vi "采配水仪器参数改变发送 (子VI).vi"(8 "错误输入":errorcluster caption="错误输出") -> (0 "错误输出":errorcluster)   [LabVIEW 2016, in "数据传输系统-03.lvlib"]
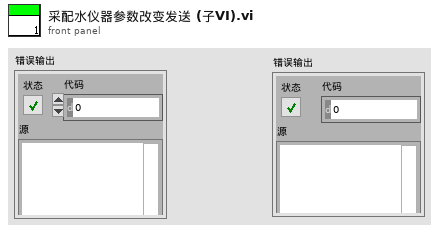
[diagram p1: front panel]
types:
  T1 = cluster{"CODMn关键参数":bool, "氨氮关键参数":bool, "总磷关键参数":bool, "总氮关键参数":bool, "CODCr关键参数":bool, "采配水关键参数":bool}
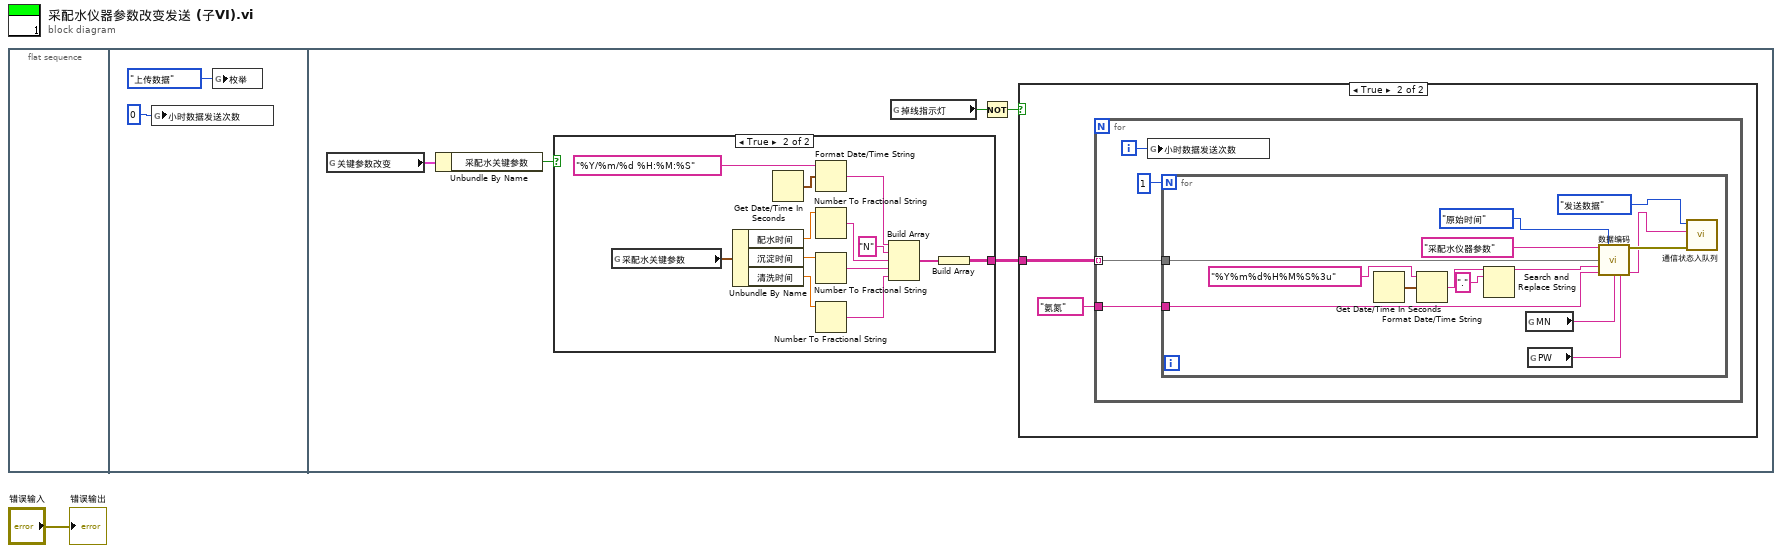
[diagram p0: block diagram]
diagram:
  n1 = flat-sequence {
    frame #0 {
    }
    frame #1 {
      n2 = global write "全局 小时数据发送次数.vi" "小时数据发送次数"(0 ("小时数据发送次数")) -> ()
      n3 = global write "全局1.vi" "枚举"(enum16{"返回请求应答", "上传数据", "返回执行结果"}."上传数据" ("枚举")) -> ()
    }
    frame #2 {
      n4 = global read "全局1.vi" "关键参数改变"() -> (w6:T1)
      n5 = Unbundle By Name(w6) -> ("采配水关键参数"=w5:bool)
      n6 = case shown="True" w5 {
        tunnel: [_ w9] -> w4
        frame False {
        }
        frame True {
          n7 = global read "全局1.vi" "采配水关键参数"() -> (w21:cluster{"配水时间":dbl, "沉淀时间":dbl, "清洗时间":dbl})
          n8 = Unbundle By Name(w21) -> ("配水时间"=w20:dbl, "沉淀时间"=w19:dbl, "清洗时间"=w18:dbl)
          n9 = Get Date/Time In Seconds() -> (seconds since 1Jan1904=w12:timestamp)
          n10 = Format Date/Time String(time format string (%c)="%Y/%m/%d %H:%M:%S" ("时间格式字符串(%c)"), seconds (now)=w12) -> (date/time string=w10:string)  [unwired: 1 in]
          n11 = Number To Fractional String(number=w20) -> (F-format string=w16:string)  [unwired: 3 in]
          n12 = Number To Fractional String(number=w19) -> (F-format string=w15:string)  [unwired: 3 in]
          n13 = Number To Fractional String(number=w18) -> (F-format string=w14:string)  [unwired: 3 in]
          n14 = Build Array(w10, "N", w16, w15, w14) -> (w17:string[])
          n15 = Build Array(w17) -> (w9:string[][])
        }
      }
      n16 = global read "全局 数据发送重叠.vi" "掉线指示灯"() -> (w8:bool)
      n17 = Not(x=w8) -> (.not. x?=w7:bool)
      n18 = case shown="True" w7 {
        tunnel: w4 -> [_ w22]
        frame False {
        }
        frame True {
          n19 = for {
            tunnel: "氨氮" ("污染物编码") -> [w27]
            tunnel: w22 -> [w26] mode=indexing
            i -> [w25]
            n20 = global write "全局 小时数据发送次数.vi" "小时数据发送次数"(w25) -> ()
            n21 = for {
              N: 1 -> [_]
              tunnel: w27 -> [w32]
              tunnel: w26 -> [w31]
              n22 = Get Date/Time In Seconds() -> (seconds since 1Jan1904=w39:timestamp)
              n23 = Format Date/Time String(time format string (%c)="%Y%m%d%H%M%S%3u" ("时间格式字符串(%c)"), seconds (now)=w39) -> (date/time string=w38:string)  [unwired: 1 in]
              n24 = Search and Replace String(input string=w38, search string="." ("搜索字符串")) -> (result string=w36:string)  [unwired: 6 in, 3 out]
              n25 = global read "断电保存全局.vi" "MN"() -> (w35:string)
              n26 = global read "断电保存全局.vi" "PW"() -> (w34:string)
              n27 = call "数据编码.vi"("table输入"="采配水仪器参数" ("新元素/子数组"), "仪器参数上传时间"=enum16{"精确到小时", "原始时间"}."原始时间", "仪器参数"=w31, "QN"=w36, "参数"=w32, "MN"=w35, "PW"=w34) -> ("错误常量"=w33:errorcluster, "通讯包字符串"=w28:string)  [unwired: 7 in]
              n28 = call "通信状态入队列.vi"("错误输入（无错误）"=w33, "发送报文"=w28, "枚举"=enum16{"打开连接", "发送数据", "读取数据", "数据处理", "关闭连接"}."发送数据") -> ()  [unwired: 8 in, 1 out]
            }
          }
        }
      }
    }
  }
  "错误输出" <- "错误输入"
